vi "Remove Node by Filter RecursiveChild.vi"(9 "Filter class instructions":refnum<class "Filter.lvclass">, 10 "Node Path (parent, child)":string[](array[string]), 11 "Tree Map In":T1) -> (0 "error out":errorcluster, 2 "Keep all parents?":bool, 3 "Tree Map Out":T1)   [LabVIEW 2020, in "Blue Tree Map OpenSource.lvlib"]
uses:
  Blue Tree Map OpenSource.lvlib
  Typedefs/Tree Map.ctl
  Typedefs/Tree Map Data.ctl
  Typedefs/Tree Node Data.ctl
  Typedefs/Attribute Map.ctl
  Classes/Filter/Filter.lvclass
  <vilib>/Utility/miscctls.llb/LVMapReplaceAction.ctl
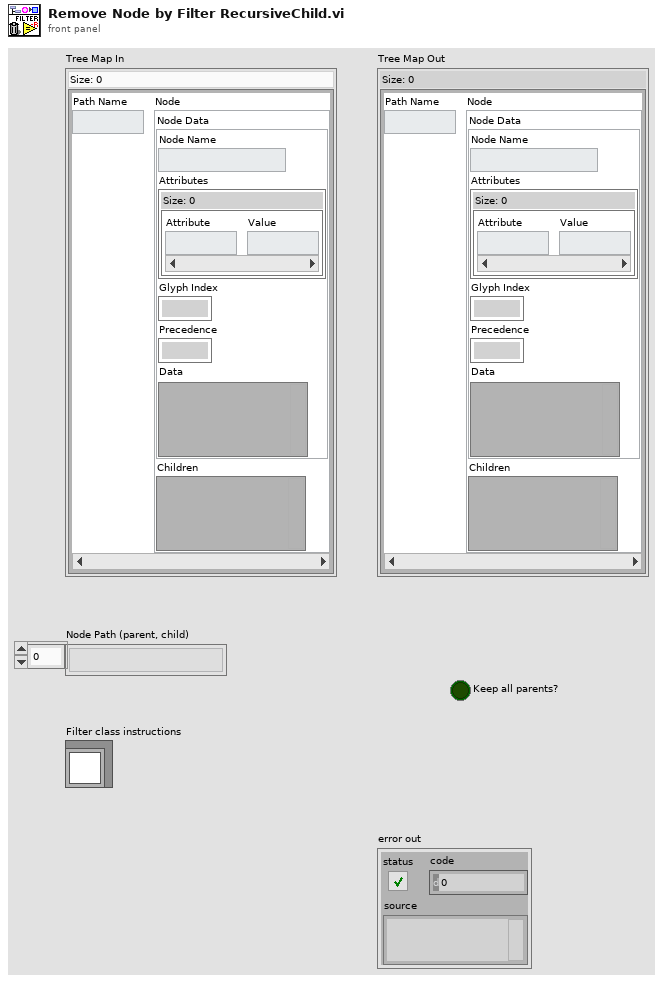
[diagram p1: front panel]
types:
  T1 = typedef "Blue Tree Map OpenSource.lvlib/Tree Map.ctl" = map{string, T2}
  T2 = typedef "Blue Tree Map OpenSource.lvlib/Tree Map Data.ctl" = cluster{"Node Data":T3, "Children":variant}
  T3 = typedef "Blue Tree Map OpenSource.lvlib/Tree Node Data.ctl" = cluster{"Node Name":string, "Attributes":T4, "Glyph Index":i32, "Precedence":i32, "Data":variant}
  T4 = typedef "Blue Tree Map OpenSource.lvlib/Attribute Map.ctl" = map{string, string}
  T5 = typedef "LVMapReplaceAction.ctl" = enum32{"Modify Entry only if found", "Add or Modify Entry", "Delete Entry"}
  T6 = typedef "Blue Tree Map OpenSource.lvlib/Filter calc option.ctl" = cluster{"Keep parents?":bool, "Keep all children?":bool}
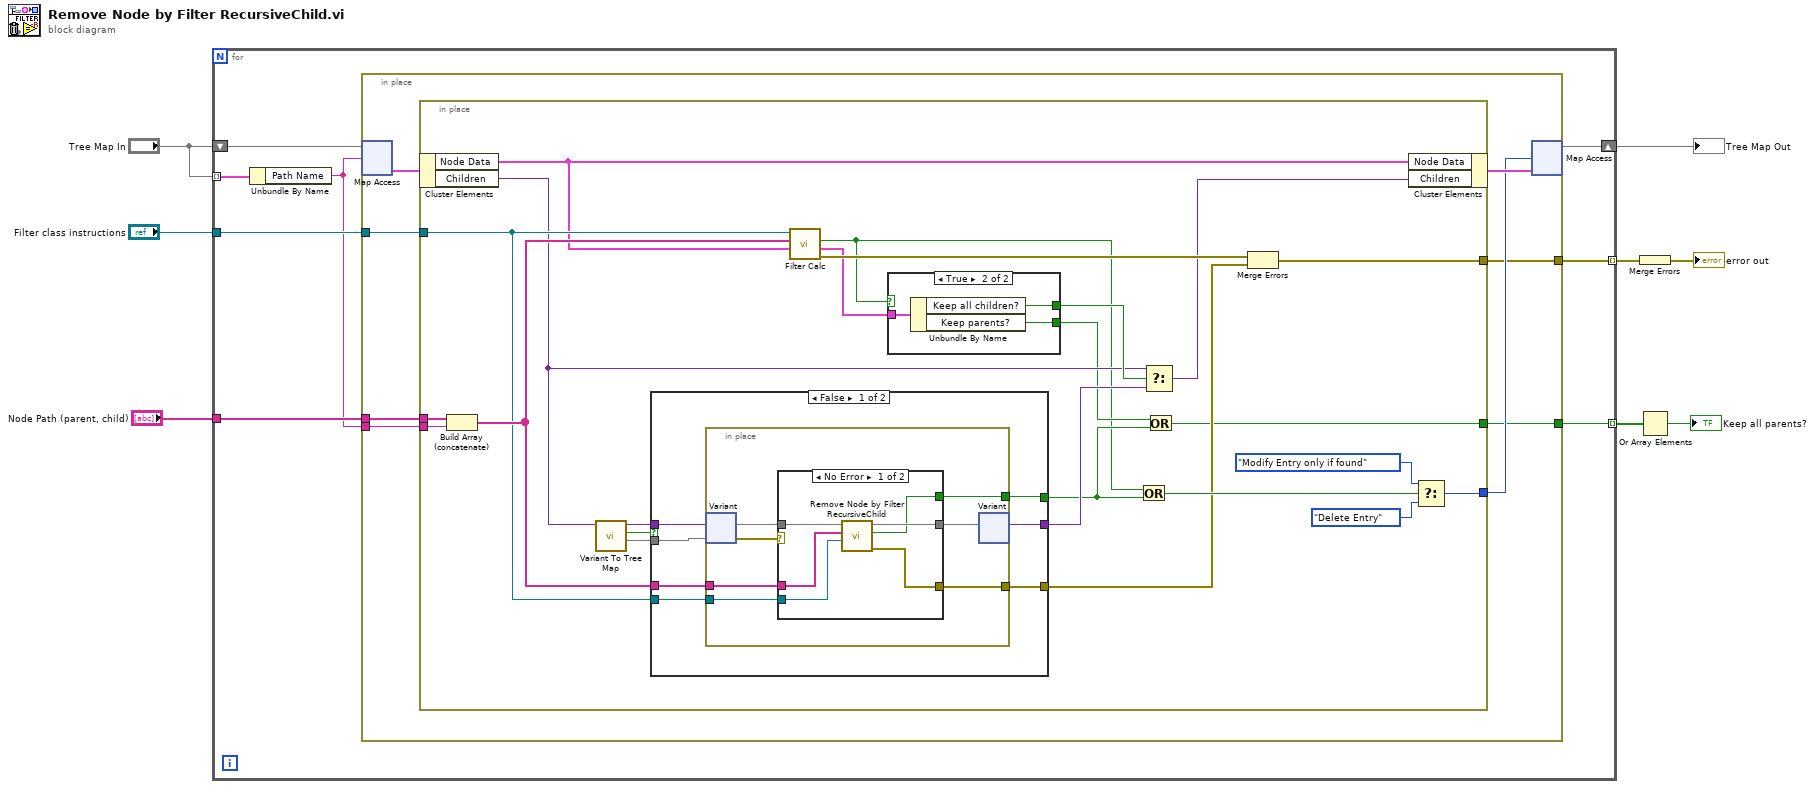
[diagram p0: block diagram]
diagram:
  n1 = for {
    tunnel: "Tree Map In" -> [w16] mode=indexing
    shift-right: [w14] -> w5
    shift-left: "Tree Map In" -> [w15]
    tunnel: "Filter class instructions" -> [w13]
    tunnel: "Node Path (parent, child)" -> [w12]
    tunnel: [w10] -> w4 mode=indexing
    tunnel: [w9] -> w2 mode=indexing
    n2 = Unbundle By Name(w16) -> ("Path Name"=w11:string)
    n3 = in-place {
      in-place-border: w13 -> [w22]
      in-place-border: w12 -> [w24]
      in-place-border: w11 -> [w23]
      in-place-border: [w18] -> w10
      in-place-border: [w17] -> w9
      n4 = in-place-map #1(w15, w11) -> (w21:T2)  [unwired: 1 in, 1 out]
      n5 = in-place {
        in-place-border: w24 -> [w48]
        in-place-border: w23 -> [w47]
        in-place-border: w22 -> [w45]
        in-place-border: [w40] -> w19
        in-place-border: [w37] -> w18
        in-place-border: [w32] -> w17
        n6 = in-place-cluster #2(w21) -> ("Node Data"=w41:T3, "Children"=w29:variant)
        n7 = Build Array (concatenate)(w48, w47) -> (w46:string[])
        n8 = call "Variant To Tree Map.vi"("Children"=w29) -> ("Tree Map (Empty)"=w33:T1, "Empty?"=w34:bool, "Children"=w35:variant)  [unwired: 8 in]
        n9 = case shown="False" w34 {
          tunnel: w46 -> [w58 _]
          tunnel: w35 -> [w57 w74]
          tunnel: w33 -> [w56 _]
          tunnel: w45 -> [w55 _]
          tunnel: [w53 w74] -> w30
          tunnel: [w54 _] -> w38
          tunnel: [w52 _] -> w26
          frame False {
            n10 = in-place {
              in-place-border: w58 -> [w65]
              in-place-border: [w64] -> w54
              in-place-border: w55 -> [w60]
              in-place-border: [w59] -> w52
              n11 = in-place-variant #3(w57, w56) -> (w63:T1, w61:errorcluster)
              n12 = case shown="No Error" w61 {
                selector: w61 -> [_ w72]
                tunnel: w65 -> [w71 _]
                tunnel: [w70 w72] -> w64
                tunnel: w63 -> [w69 w73]
                tunnel: [w68 w73] -> w62
                tunnel: w60 -> [w67 _]
                tunnel: [w66 _] -> w59
                frame No Error {
                  n13 = call "Remove Node by Filter RecursiveChild.vi"("Filter class instructions"=w67, "Node Path (parent, child)"=w71, "Tree Map In"=w69) -> ("error out"=w70:errorcluster, "Keep all parents?"=w66:bool, "Tree Map Out"=w68:T1)  [unwired: 6 in]
                }
                frame Error {
                }
              }
              n14 = in-place-variant #3(w62) -> (w53:variant)  [unwired: 1 out]
            }
          }
          frame True {
          }
        }
        n15 = call-dynamic "Filter Calc.vi"("Node Data"=w41, "Node Path (parent, child)"=w46, "Filter in"=w45) -> ("error out"=w39:errorcluster, "Keep options"=w36:T6, "Keep node?"=w25:bool)  [unwired: 5 in, 1 out]
        n16 = case shown="True" w25 {
          tunnel: w36 -> [_ w51]
          tunnel: [_ w50] -> w31
          tunnel: [_ w49] -> w27
          frame False {
          }
          frame True {
            n17 = Unbundle By Name(w51) -> ("Keep all children?"=w50:bool, "Keep parents?"=w49:bool)
          }
        }
        n18 = Or(x=w25, y=w26) -> (x .or. y?=w44:bool)
        n19 = Select(t=w29, s=w31, f=w30) -> (s? t:f=w28:variant)
        n20 = Or(x=w27, y=w26) -> (x .or. y?=w32:bool)
        n21 = Merge Errors(w39, w38) -> (w37:errorcluster)
        n22 = in-place-cluster #2("Node Data"=w41, "Children"=w28) -> (w20:T2)
        n23 = Select(t=LVMapReplaceAction."Modify Entry only if found" ("action"), s=w44, f=LVMapReplaceAction."Delete Entry" ("action")) -> (s? t:f=w40:T5)
      }
      n24 = in-place-map #1(w20, w19) -> (w14:T1)  [unwired: 2 out]
    }
  }
  "Tree Map Out" <- w5
  n25 = Merge Errors(w4) -> (→"error out":errorcluster)
  n26 = Or Array Elements(Boolean array=w2) -> (logical OR=→"Keep all parents?":bool)
